vi "Search for Subordinate.vi"(8 "error in":errorcluster, 10 "Identifier":string, 11 "Base Software in":refnum<class "Main.lvclass">) -> (0 "error out":errorcluster, 1 "Found":bool, 2 "Enqueuer":refnum<class "Message Enqueuer.lvclass">, 3 "Base Software out":refnum<class "Main.lvclass">, 4 "Index":i32, 5 "Position":T1)   [LabVIEW 2023, in "Main.lvlib" / "Main.lvclass"]
uses:
  Project/Main.lvclass
  builds/Engine/Actor Framework.lvlibp/1abvi3w/vi.lib/ActorFramework/Message Enqueuer/Message Enqueuer.lvclass
  Custom Controls/Panel_Positions.ctl
  Project/Main.lvclass/Main.ctl
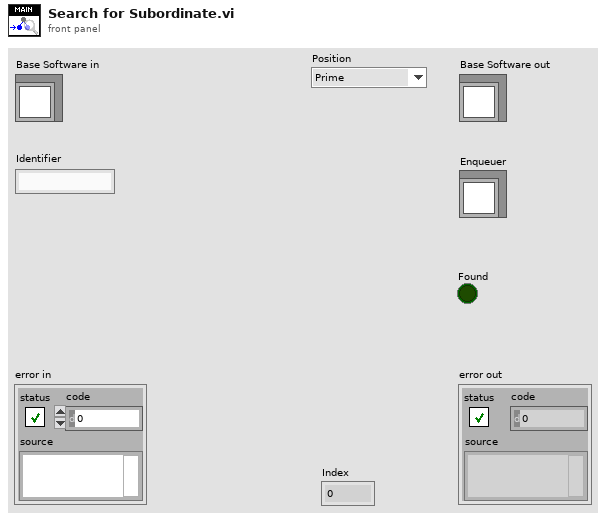
[diagram p1: front panel]
types:
  T1 = typedef "Main.lvlib/Main.lvclass/Panel_Positions.ctl" = enum16{"Prime", "Right", "Bottom", "Left", "Mission"}
  T2 = typedef "Main.lvlib/Main.lvclass/Subordinate.ctl" = cluster{"Identifier":string, "Enqueuer":refnum<class "Message Enqueuer.lvclass">, "Position":T1}
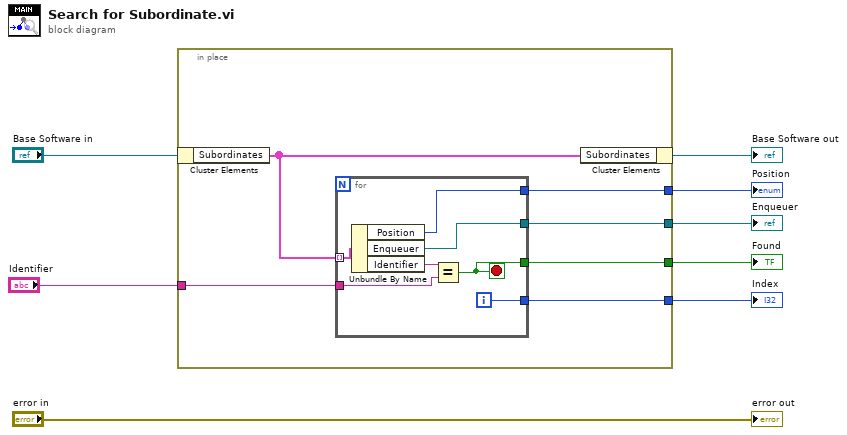
[diagram p0: block diagram]
diagram:
  n1 = in-place {
    in-place-border: "Identifier" -> [w13]
    in-place-border: [w12] -> w5
    in-place-border: [w11] -> w4
    in-place-border: [w10] -> w2
    in-place-border: [w9] -> w1
    n2 = in-place-cluster #1("Base Software in") -> ("Subordinates"=w14:T2[])
    n3 = for {
      tunnel: w14 -> [w21] mode=indexing
      tunnel: w13 -> [w19]
      tunnel: [w18] -> w12
      tunnel: [w17] -> w11
      tunnel: [w16] -> w10
      tunnel: [w15] -> w9
      i -> [w17]
      stop <- w18 stop-if-true
      n4 = Unbundle By Name(w21) -> ("Position"=w15:T1, "Enqueuer"=w16:refnum<class "Message Enqueuer.lvclass">, "Identifier"=w20:string)
      n5 = Equal?(x=w20, y=w19) -> (x = y?=w18:bool)
    }
    n6 = in-place-cluster #1("Subordinates"=w14) -> (→"Base Software out":refnum<class "Main.lvclass">)
  }
  "Found" <- w5
  "Index" <- w4
  "Enqueuer" <- w2
  "Position" <- w1
  "error out" <- "error in"
